vi "Write off2.vi"(8 "error in (no error)":errorcluster, 10 "off2":dbl[unit] min=-0.00048481368110953597 max=0.00048481368110953597, 11 "OffsetStatus in":refnum<class "OffsetStatus.lvclass">) -> (0 "error out":errorcluster, 3 "OffsetStatus out":refnum<class "OffsetStatus.lvclass">)   [LabVIEW 2014]
uses:
  OffsetStatus.lvclass
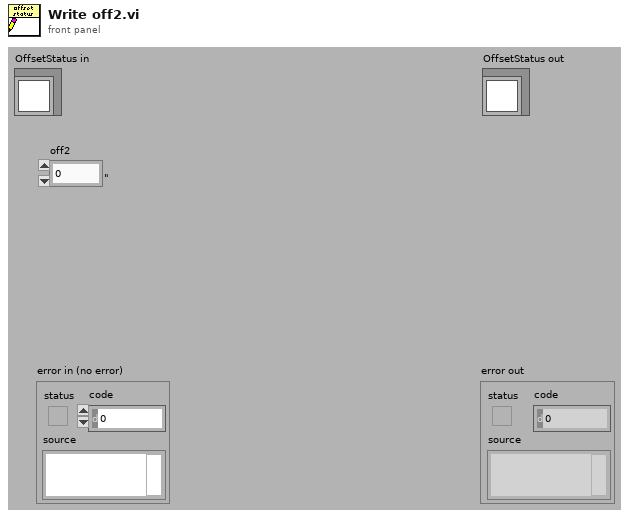
[diagram p1: front panel]
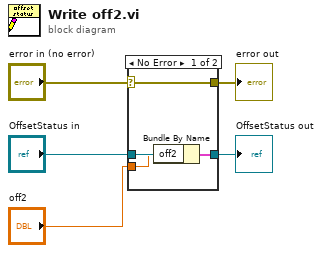
[diagram p0: block diagram]
diagram:
  n1 = case shown="No Error" "error in (no error)" {
    selector: "error in (no error)" -> [w9 w10]
    tunnel: [w9 w10] -> w4
    tunnel: [w7 w11] -> w1
    tunnel: "OffsetStatus in" -> [w8 w11]
    tunnel: "off2" -> [w6 _]
    frame No Error {
      n2 = Bundle By Name(cluster=w8, "off2"=w6) -> (w7:cluster{})
    }
    frame Error {
    }
  }
  "error out" <- w4
  "OffsetStatus out" <- w1
